vi "utility.DelayTime.Window.vi"(11 "Timer":dbl min=0.0 step=0.01) -> ()   [LabVIEW 2012, in "Lib_UEL.ATE.lvlib" / "Lib_App.lvlib"]
uses:
  Lib_App.lvlib
panel:
  out "错误输出":errorcluster
  out "TimerMeter":dbl(knob)=2.7755575615628914e-17 scale=0.0..10.0
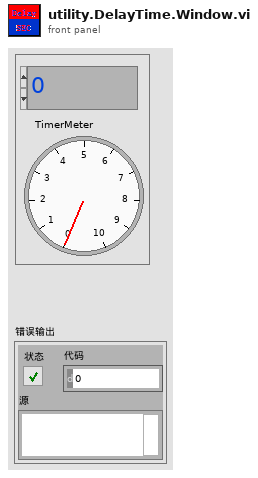
[diagram p1: front panel]
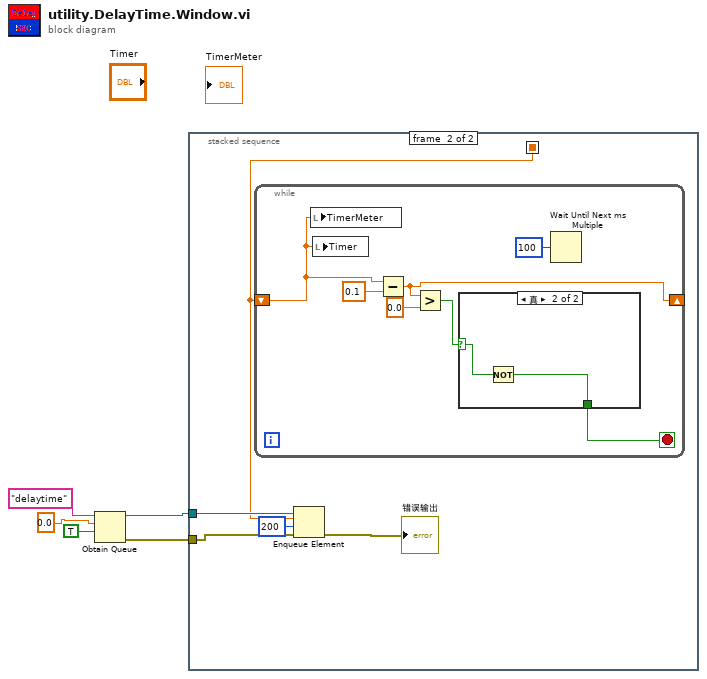
[diagram p0: block diagram]
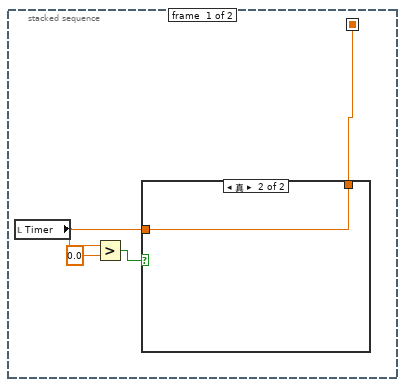
[diagram p2: hidden frame]
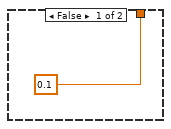
[diagram p3: hidden frame]
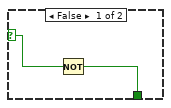
[diagram p4: hidden frame]
diagram:
  n1 = Obtain Queue(name (unnamed)="delaytime" ("名称（未命名）"), element data type=0.0 ("y"), create if not found? (T)=TRUE ("如未找到是否创建？(T)")) -> (queue out=w2:refnum<queue>, error out=w1:errorcluster)  [unwired: 2 in, 1 out]
  n2 = stacked-sequence {
    seq-local: [w7 _] -> [_ w14]
    tunnel: w2 -> [_ w16]
    tunnel: w1 -> [_ w15]
    frame #0 {
      n3 = local read "Timer"() -> (w6:dbl)
      n4 = Greater?(x=w6, y=0.0) -> (0:w8:bool)
      n5 = case shown="真" w8 {
        tunnel: [0.1 ("Timer") w11] -> w7
        tunnel: w6 -> [_ w11]
        frame False {
        }
        frame True {
        }
      }
    }
    frame #1 {
      n6 = while {
        shift-right: [w21] -> _
        shift-left: w14 -> [w18]
        stop <- w19 stop-if-true
        n7 = local write "TimerMeter"(w18) -> ()
        n8 = local write "Timer"(w18) -> ()
        n9 = Subtract(x=w18, y=0.1) -> (x-y=w21:dbl)
        n10 = Greater?(x=w21, y=0.0) -> (0:w20:bool)
        n11 = case shown="真" w20 {
          selector: w20 -> [w25 w27]
          tunnel: [w24 w26] -> w19
          frame False {
            n12 = Not(x=w25) -> (.not. x?=w24:bool)
          }
          frame True {
            n13 = Not(x=w27) -> (.not. x?=w26:bool)
          }
        }
        n14 = Wait Until Next ms Multiple(millisecond multiple=u32 100 ("毫秒倍数")) -> ()  [unwired: 1 out]
      }
      n15 = Enqueue Element(queue=w16, element=w14, timeout in ms (-1)=200 ("超时毫秒(-1)"), error in (no error)=w15) -> (error out=→"错误输出":errorcluster)  [unwired: 2 out]
    }
  }
